vi "ShowErrors Dialog.vi"(8 "error in (no error)":errorcluster, 9 "ErrorList":string[](array[string]), 10 "menubar":refnum<k9>, 11 "Main UI Ref":refnum<vi>) -> (0 "error out":errorcluster)   [LabVIEW 2017, in "ErrorHandler.lvclass"]
doc: "Developed by Kevin Thompson\nkevin@thompsonengineering.net\n\nCopyright 2018\nThompson Engineering, LLC"
uses:
  ErrorHandler.lvclass
  ErrorHandler.lvclass/ErrorHandler.ctl
  Accessors/Get ErrorList Qref.vi
panel:
  out "ErrorList out":string[](array[string]) caption="Errors"
  in  "Close":bool
  in  "ClearErrorList":bool
  # "Error List"
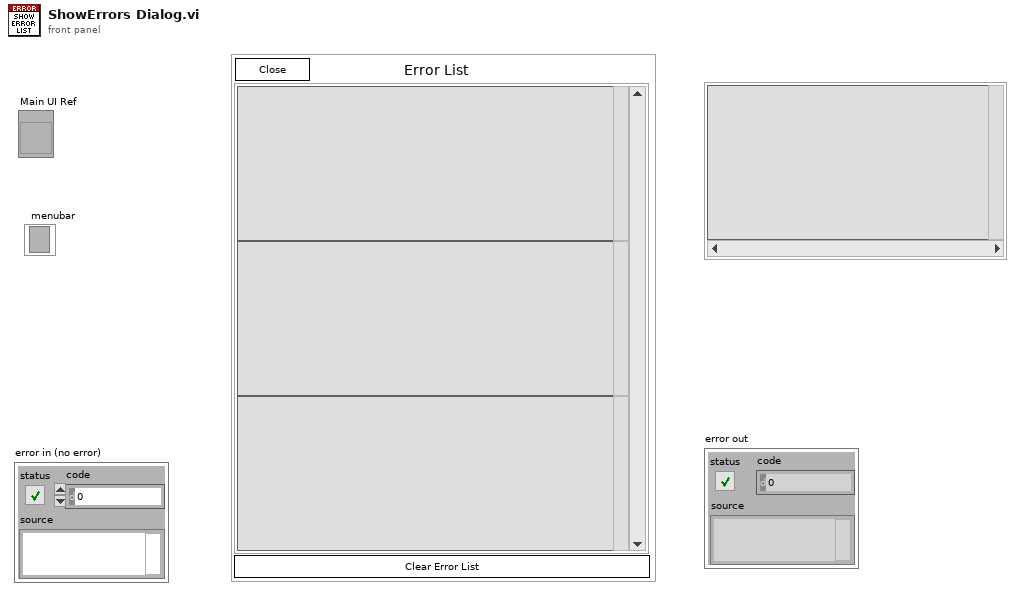
[diagram p1: front panel]
types:
  T1 = enum32{"Invalid", "Default", "Floating", "Floating/Auto-Hide", "Modal"}
  T2 = enum32{"Invalid", "Standard", "Closed", "Hidden", "Minimized", "Maximized"}
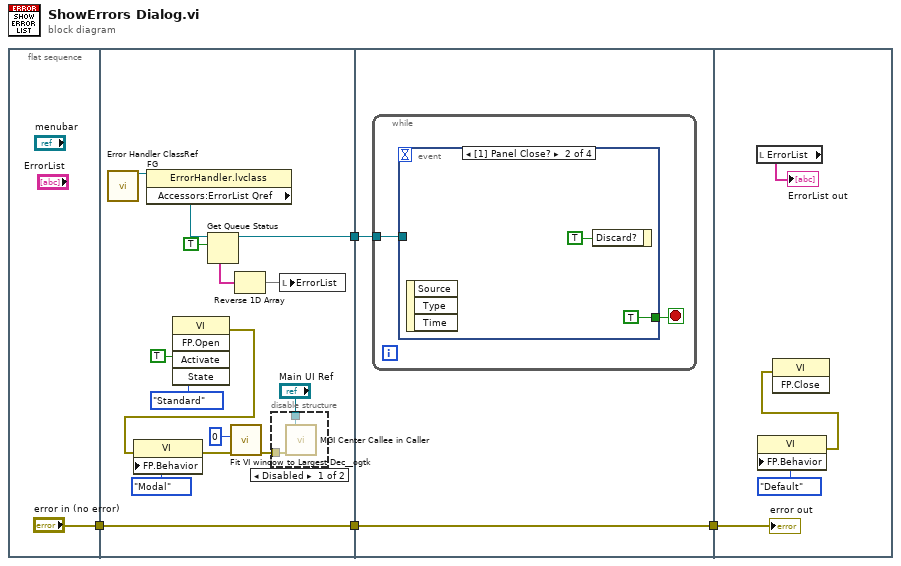
[diagram p0: block diagram]
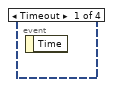
[diagram p3: hidden frame]
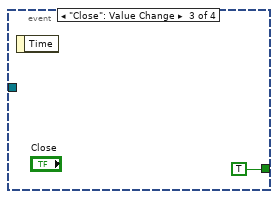
[diagram p4: hidden frame]
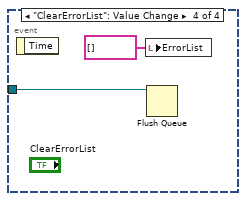
[diagram p5: hidden frame]
diagram:
  n1 = flat-sequence {
    tunnel: ["error in (no error)"] -> w3
    tunnel: [w11] -> w4
    tunnel: w3 -> [w11]
    tunnel: [w9] -> w1
    tunnel: w4 -> [w24]
    tunnel: [w24] -> w2
    tunnel: w1 -> [w23]
    tunnel: w2 -> [w32]
    frame #0 {
    }
    frame #1 {
      n2 = call "Error Handler ClassRef FG.vi"() -> ("ErrorHandler out"=w8:refnum<class "ErrorHandler.lvclass">)  [unwired: 10 in, 1 out]
      n3 = property class="ErrorHandler.lvclass"(reference=w8) -> ("Accessors:ErrorList Qref"=w7:refnum<queue>)  [unwired: 1 in, 2 out]
      n4 = invoke class="VI" method="FP.Open"("Activate"=TRUE ("Activate?"), "State"=T2."Standard") -> (error out=w17:errorcluster)  [unwired: 3 in, 4 out]
      n5 = property class="VI"(error in=w17, "FP.Behavior"=T1."Modal" ("Front Panel Window:Behavior")) -> (error out=w16:errorcluster)  [unwired: 1 in, 1 out]
      n6 = Get Queue Status(queue=w7, return elements? (F)=TRUE) -> (queue out=w9:refnum<queue>, elements=w10:string[])  [unwired: 1 in, 6 out]
      n7 = call <userlib>:"Fit VI window to Largest Dec__ogtk.vi"("error in (no error)"=w16, "border spacing (2 px)"=0) -> ("error out"=w14:errorcluster)  [unwired: 4 in, 1 out]
      n8 = Reverse 1D Array(array=w10) -> (reversed array=w6:string[])
      n9 = disable-structure shown="Disabled" {
        disable-tunnel: w14 -> [w22 _]
        disable-tunnel: "Main UI Ref" -> [w21 _]
        frame Disabled {
          n10 = call <userlib>:"MGI Center Callee in Caller.vi"("Error In"=w22, "Caller VI Refnum (Callee's Caller)"=w21) -> ()  [unwired: 9 in, 1 out]
        }
        frame Enabled {
        }
      }
      n11 = local write "ErrorList"(w6) -> ()
    }
    frame #2 {
      n12 = while {
        tunnel: w23 -> [w25]
        stop <- w26 stop-if-true
        n13 = event shown="[1] Panel Close?" {
          selector: _ -> [_ _ _ _]
          dyn-events: _ -> [_ _ _ _]
          timeout: _ -> [_ _ _ _]
          tunnel: [_ TRUE TRUE _] -> w26
          tunnel: w25 -> [_ _ _ w30]
          event Timeout {
            n14 = event-data() -> ()  [unwired: 1 in, 1 out]
          }
          event Panel Close? {
            n15 = event-data() -> ()  [unwired: 1 in, 3 out]
            n16 = event-data("Discard?"=TRUE) -> ()  [unwired: 1 in, 1 out]
          }
          event "Close": Value Change {
            n17 = event-data() -> ()  [unwired: 1 in, 1 out]
          }
          event "ClearErrorList": Value Change {
            n18 = event-data() -> ()  [unwired: 1 in, 1 out]
            n19 = local write "ErrorList"(string[] [] ("ErrorList")) -> ()
            n20 = Flush Queue(queue=w30) -> ()  [unwired: 1 in, 3 out]
          }
        }
      }
    }
    frame #3 {
      n21 = local read "ErrorList"() -> (→"ErrorList out":string[])
      n22 = property class="VI"("FP.Behavior"=T1."Default" ("Front Panel Window:Behavior")) -> (error out=w34:errorcluster)  [unwired: 2 in, 1 out]
      n23 = invoke class="VI" method="FP.Close"(error in=w34) -> ()  [unwired: 2 in, 3 out]
      "error out" <- w32
    }
  }
